vi "Apply.vi"(8 "error in":errorcluster, 11 "DO DAQmx Fixed Freq PWM CFG in":refnum<class "DO DAQmx Fixed Freq PWM CFG.lvclass">) -> (0 "error out":errorcluster, 3 "DO DAQmx Fixed Freq PWM CFG out":refnum<class "DO DAQmx Fixed Freq PWM CFG.lvclass">)   [LabVIEW 2023, in "DO DAQmx Fixed Freq PWM CFG.lvclass"]
uses:
  DO DAQmx Fixed Freq PWM CFG.lvclass
  DO DAQmx Fixed Freq PWM CFG.lvclass/DO DAQmx Fixed Freq PWM CFG.ctl
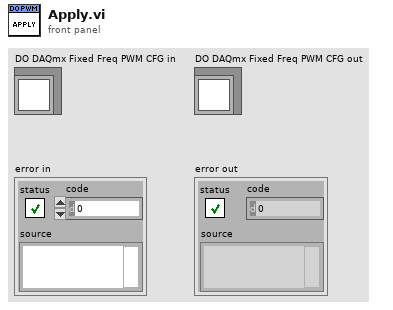
[diagram p1: front panel]
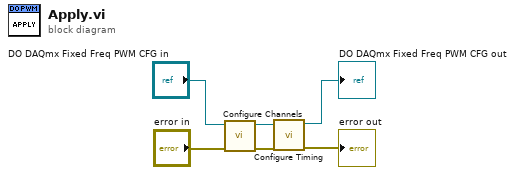
[diagram p0: block diagram]
diagram:
  n1 = call-dynamic "Configure Channels.vi"("error in"="error in", "DO DAQmx Fixed Freq PWM CFG in"="DO DAQmx Fixed Freq PWM CFG in") -> ("error out"=w5:errorcluster, "DO DAQmx Fixed Freq PWM CFG out"=w6:refnum<class "DO DAQmx Fixed Freq PWM CFG.lvclass">)  [unwired: 8 in]
  n2 = call-dynamic "Configure Timing.vi"("error in (no error)"=w5, "DAQmx Base CFG in"=w6) -> ("error out"=→"error out":errorcluster, "DAQmx Base CFG out"=→"DO DAQmx Fixed Freq PWM CFG out":refnum<class "DO DAQmx Fixed Freq PWM CFG.lvclass">)  [unwired: 8 in]
